vi "Ask for mm Distance.vi"() -> (3 "distance (mm) out":dbl=1.0)   [LabVIEW 2020]
panel:
  in  "continue":bool
  in  "distance (mm)":dbl=1.0
  # "How many millimeters does the line correspond to?"
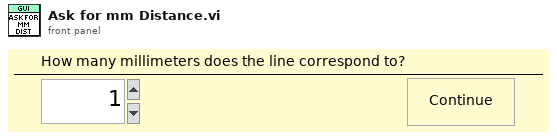
[diagram p1: front panel]
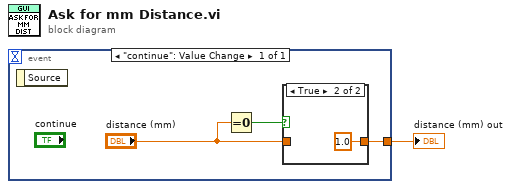
[diagram p0: block diagram]
diagram:
  n1 = event shown="[0] \"continue\": Value Change" {
    selector: _ -> [_]
    dyn-events: _ -> [_]
    timeout: _ -> [_]
    tunnel: [w3] -> w1
    event "continue": Value Change {
      n2 = event-data() -> ()  [unwired: 1 in, 1 out]
      n3 = Equal To 0?(x="distance (mm)") -> (x = 0?=w4:bool)
      n4 = case shown="True" w4 {
        tunnel: [w5 1.0 ("distance (mm)")] -> w3
        tunnel: "distance (mm)" -> [w5 _]
        frame False {
        }
        frame True {
        }
      }
    }
  }
  "distance (mm) out" <- w1
